vi "CRYScale Wave.vi"(5 "Level Type":u16, 7 "EQGain":dbl, 8 "Level":sgl format="%#_6p", 9 "dB ref":dbl format="%#_6p", 10 "Max":dbl, 11 "Wave":sgl[](array[numeric])) -> (1 "Max Out":sgl format="%#_6p", 2 "Crest Factor":sgl, 3 "Scaled Wave":sgl[](array[numeric]))   [LabVIEW 2013]
uses:
  <vilib>/Analysis/5stat.llb/RMS (DBL).vi
  <vilib>/Analysis/NI_AALPro.lvlib
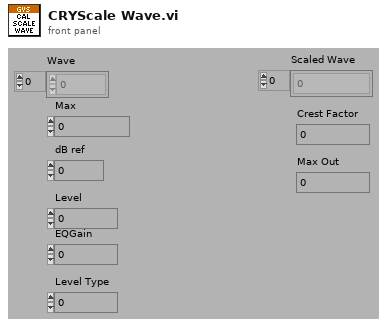
[diagram p1: front panel]
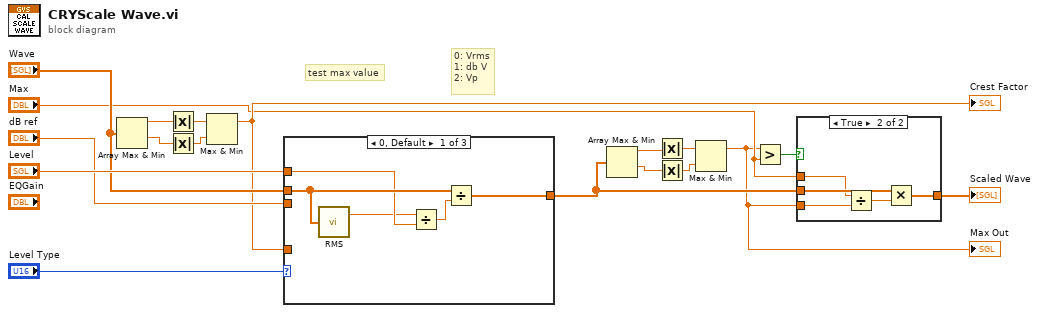
[diagram p0: block diagram]
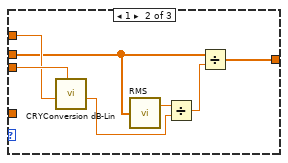
[diagram p3: hidden frame]
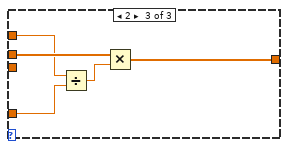
[diagram p4: hidden frame]
diagram:
  # "test max value"
  # "0: Vrms\n1: db V\n2: Vp"
  n1 = Array Max & Min(array="Wave") -> (max value=w16:sgl, min value=w15:sgl)  [unwired: 2 out]
  n2 = Absolute Value(x=w16) -> (abs(x)=w14:sgl)
  n3 = Absolute Value(x=w15) -> (abs(x)=w13:sgl)
  n4 = Max & Min(x=w14, y=w13) -> (max(x,y)=w10:sgl)  [unwired: 1 out]
  "Crest Factor" <- w10
  n5 = case shown="0, Default" "Level Type" {
    tunnel: w10 -> [_ _ w32]
    tunnel: "Level" -> [w21 w28 w33]
    tunnel: "dB ref" -> [_ w30 _]
    tunnel: "Wave" -> [w23 w27 w35]
    tunnel: [w22 w29 w34] -> w4
    frame 0, Default {
      n6 = call-poly <vilib>:"RMS.vi"("X"=w23) -> ("rms value"=w20:dbl)  [unwired: 1 out]
      n7 = Divide(x=w20, y=w21) -> (x/y=w19:dbl)
      n8 = Divide(x=w23, y=w19) -> (x/y=w22:dbl[])
    }
    frame 1 {
      n9 = call "CRYConversion dB-Lin.vi"("dB ref."=w30, "Log In"=w28) -> ("Lin Out"=w24:dbl)  [unwired: 4 in, 3 out]
      n10 = call-poly <vilib>:"RMS.vi"("X"=w27) -> ("rms value"=w26:dbl)  [unwired: 1 out]
      n11 = Divide(x=w26, y=w24) -> (x/y=w25:dbl)
      n12 = Divide(x=w27, y=w25) -> (x/y=w29:dbl[])
    }
    frame 2 {
      n13 = Divide(x=w33, y=w32) -> (x/y=w31:sgl)
      n14 = Multiply(x=w35, y=w31) -> (x*y=w34:sgl[])
    }
  }
  n15 = Array Max & Min(array=w4) -> (max value=w7:dbl, min value=w6:dbl)  [unwired: 2 out]
  n16 = Absolute Value(x=w7) -> (abs(x)=w8:dbl)
  n17 = Absolute Value(x=w6) -> (abs(x)=w9:dbl)
  n18 = Max & Min(x=w8, y=w9) -> (max(x,y)=w1:dbl)  [unwired: 1 out]
  "Max Out" <- w1
  n19 = Greater?(x=w1, y="Max") -> (0:w5:bool)
  n20 = case shown="True" w5 {
    tunnel: w4 -> [w36 w40]
    tunnel: [w36 w41] -> w3
    tunnel: w1 -> [_ w38]
    tunnel: "Max" -> [_ w37]
    frame False {
    }
    frame True {
      n21 = Divide(x=w37, y=w38) -> (x/y=w39:dbl)
      n22 = Multiply(x=w40, y=w39) -> (x*y=w41:dbl[])
    }
  }
  "Scaled Wave" <- w3
